vi "SHA256.vi"() -> ()   [LabVIEW 2019]
panel:
  out "hmac_str 2":string
  out "length":i32
  out "x = y?":bool
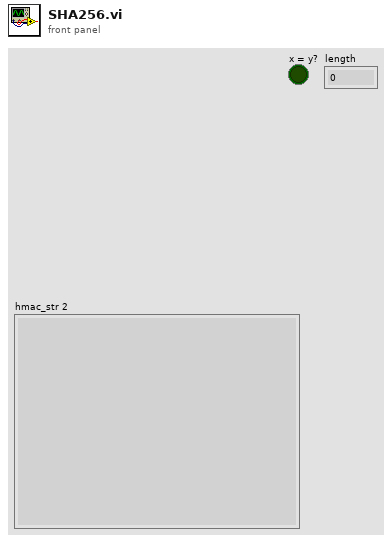
[diagram p1: front panel]
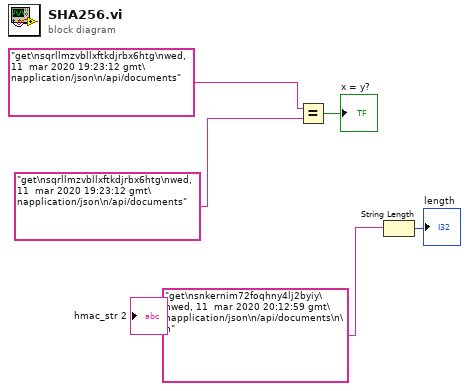
[diagram p0: block diagram]
diagram:
  n1 = Equal?(x="get\nsqrllmzvbllxftkdjrbx6htg\nwed, 11  mar 2020 19:23:12 gmt\napplication/json\n/api/documents", y="get\nsqrllmzvbllxftkdjrbx6htg\nwed, 11  mar 2020 19:23:12 gmt\napplication/json\n/api/documents") -> (x = y?=→"x = y?":bool)
  n2 = String Length(string="get\nsnkernim72foqhny4lj2byiy\nwed, 11  mar 2020 20:12:59 gmt\napplication/json\n/api/documents\n\n" ("hmac_str")) -> (length=→"length":i32)
